vi "test Add-Import-Deploy.vi"(8 "error in":errorcluster, 11 "Import-Script-Deploy.lvclass":refnum<class "Import-Script-Deploy.lvclass">) -> (0 "error out":errorcluster, 3 "Import-Script-Deploy.lvclass":refnum<class "Import-Script-Deploy.lvclass">)   [LabVIEW 2020, in "Import-Script-Deploy.lvclass"]
uses:
  Import-Script-Deploy.lvclass
  C:/Git/niveristand-custom-device-testing-tools/VeriStandTestCase/VeriStandTestCase.lvclass
  Shared/Device Parameters.ctl
  Shared/Initialization Method.ctl
  Import-Script-Deploy.lvclass/Import-Script-Deploy.ctl
  4b06c685-66bb-4135-9ad1-d89a50a95502.vi
  <vilib>/addons/_JKI Toolkits/VI Tester/TestCase.llb/TestCase.lvclass
  Scripting/Ballard/Ballard ARINC 429 Scripting.lvlib
  niveristand-custom-device-testing-tools/VeriStandTestUtilities/VeriStandTestUtilities.lvlib
  C:/Program Files (x86)/National Instruments/LabVIEW 2020/vi.lib/addons/_JKI Toolkits/VI Tester/TestCase.llb/TestCase.lvclass
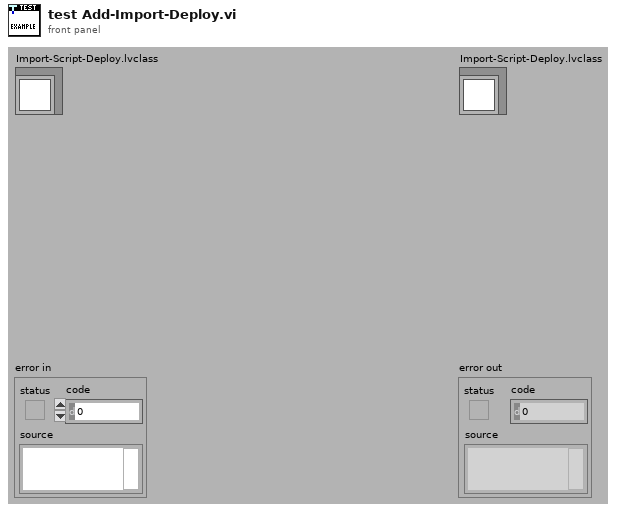
[diagram p1: front panel]
types:
  T1 = typedef "Device Parameters.ctl" = cluster{"initialization method":T2, "card number":i32, "PXI slot number":i32, "core number":i32}
  T2 = typedef "Initialization Method.ctl" = enum16{"PXI Slot Number", "Card Number"}
  T3 = typedef "Custom Device API.lvlib/Custom Device Item Ref.ctl" = u64
  T4 = typedef "NI_VS Workspace ExecutionAPI.lvlib/WorkspaceAPI.ctl" = refnum<k24>
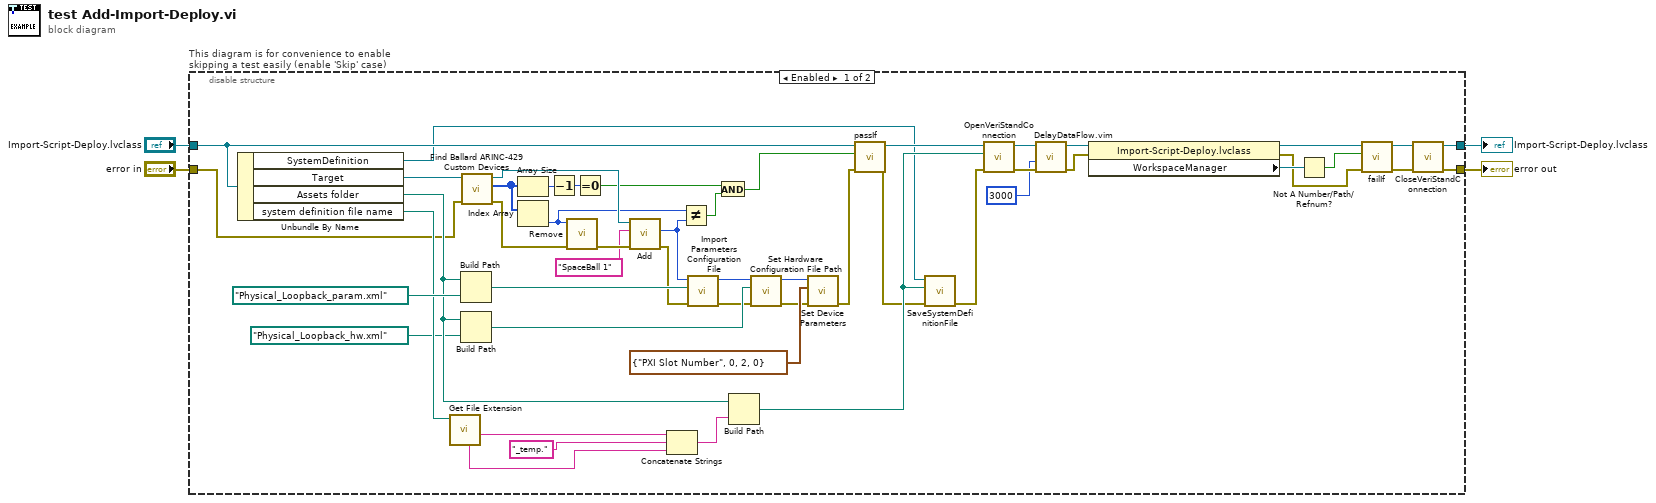
[diagram p0: block diagram]
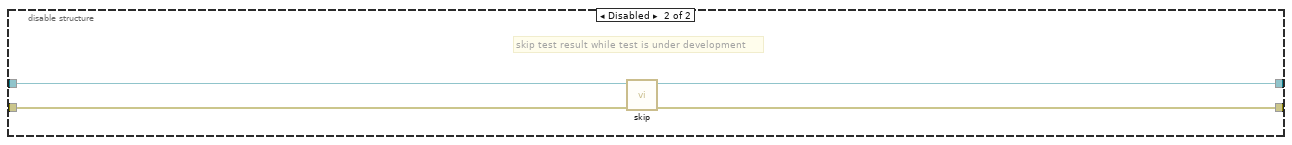
[diagram p2: hidden frame]
diagram:
  n1 = disable-structure "This diagram is for convenience to enable skipping a test easily (enable 'Skip' case)" shown="Enabled" {
    disable-tunnel: "Import-Script-Deploy.lvclass" -> [w43 w57]
    disable-tunnel: [w52 w56] -> w3
    disable-tunnel: "error in" -> [w21 w55]
    disable-tunnel: [w45 w54] -> w1
    frame Enabled {
      n2 = Unbundle By Name(w43) -> ("SystemDefinition"=w22:refnum<k24>, "Target"=w44:refnum<k24>, "Assets folder"=w28:path, "system definition file name"=w36:path)
      n3 = call <vilib>:"Get File Extension.vi"("file"=w36) -> ("filename without extension"=w35:string, "unmodified file extension"=w33:string)  [unwired: 6 in, 3 out]
      n4 = Build Path(base path=w28, name or relative path=path "Physical_Loopback_param.xml" ("Absolute or Relative Path")) -> (appended path=w18:path)
      n5 = Build Path(base path=w28, name or relative path=path "Physical_Loopback_hw.xml" ("Absolute or Relative Path")) -> (appended path=w26:path)
      n6 = call "Find Ballard ARINC-429 Custom Devices.vi"("error in"=w21, "target in"=w44) -> ("error out"=w13:errorcluster, "Ballard ARINC 429 custom devices"=w20:u64[], "target out"=w15:refnum<k24>)  [unwired: 7 in]
      n7 = Array Size(array=w20) -> (size(s)=w11:i32)
      n8 = Index Array(array=w20) -> (element=w8:u64)  [unwired: 1 in]
      n9 = Decrement(x=w11) -> (x-1=w10:i32)
      n10 = call "Remove.vi"("error in"=w13, "Ballard ARINC 429 custom device"=w8) -> ("error out"=w16:errorcluster)  [unwired: 9 in]
      n11 = Equal To 0?(x=w10) -> (x = 0?=w7:bool)
      n12 = call "Add.vi"("error in"=w16, "name"="SpaceBall 1", "target in"=w15) -> ("error out"=w12:errorcluster, "Ballard ARINC 429 ref out"=w9:T3)  [unwired: 6 in, 1 out]
      n13 = Concatenate Strings(w35, "_temp." ("string"), w33) -> (w32:string)
      n14 = Not Equal?(x=w8, y=w9) -> (x != y?=w6:bool)
      n15 = call "Import Parameters Configuration File.vi"("error in"=w12, "parameters configuration file path"=w18, "Ballard ARINC 429 ref"=w9) -> ("error out"=w17:errorcluster, "Ballard ARINC 429 ref out"=w19:T3)  [unwired: 7 in]
      n16 = And(x=w7, y=w6) -> (x .and. y?=w5:bool)
      n17 = Build Path(base path=w28, name or relative path=w32) -> (appended path=w31:path)
      n18 = call "Set Hardware Configuration File Path.vi"("error in"=w17, "path"=w26, "custom device ref"=w19) -> ("error out"=w24:errorcluster, "custom device ref out"=w25:T3)  [unwired: 7 in]
      n19 = call "Set Device Parameters.vi"("error in"=w24, "device parameters"=T1 {"initialization method"=enum."PXI Slot Number", "card number"=0, "PXI slot number"=2, "core number"=0}, "Ballard ARINC 429 custom device in"=w25) -> ("error out"=w23:errorcluster)  [unwired: 7 in, 1 out]
      n20 = call-dynamic "passIf.vi"("error in (no error)"=w23, "pass"=w5, "TestCase in"=w43) -> ("error out"=w29:errorcluster, "TestCase out"=w42:refnum<class "Import-Script-Deploy.lvclass">)  [unwired: 7 in]
      n21 = call "SaveSystemDefinitionFile.vi"("error in (no error)"=w29, "System Definition File in"=w31, "System Definition Reference in"=w22) -> ("error out"=w30:errorcluster)  [unwired: 7 in, 1 out]
      n22 = call-dynamic "OpenVeriStandConnection.vi"("error in (no error)"=w30, "System Definition File"=w31, "VeriStand Test Case in"=w42) -> ("error out"=w41:errorcluster, "VeriStand Test Case out"=w40:refnum<class "Import-Script-Deploy.lvclass">)  [unwired: 6 in, 1 out]
      n23 = call "DelayDataFlow.vim"("value in"=w41, "milliseconds to wait"=u32 3000) -> ("value out"=w53:errorcluster)  [unwired: 2 in, 1 out]
      n24 = property class="Import-Script-Deploy.lvclass"(reference=w40, error in=w53) -> (reference out=w51:refnum<class "Import-Script-Deploy.lvclass">, error out=w46:errorcluster, "WorkspaceManager"=w48:T4)
      n25 = Not A Number/Path/Refnum?(number/path/refnum=w48) -> (NaN/Path/Refnum?=w47:bool)
      n26 = call-dynamic "failIf.vi"("error in (no error)"=w46, "fail"=w47, "TestCase in"=w51) -> ("error out"=w49:errorcluster, "TestCase out"=w50:refnum<class "Import-Script-Deploy.lvclass">)  [unwired: 7 in]
      n27 = call-dynamic "CloseVeriStandConnection.vi"("error in (no error)"=w49, "VeriStand Test Case in"=w50) -> ("error out"=w52:errorcluster, "VeriStand Test Case out"=w45:refnum<class "Import-Script-Deploy.lvclass">)  [unwired: 8 in]
    }
    frame Disabled {
      # "skip test result while test is under development"
      n28 = call <vilib>:"skip.vi"("error in (no error)"=w55, "TestCase in"=w57) -> ("error out"=w56:errorcluster, "TestCase out"=w54:refnum<class "Import-Script-Deploy.lvclass">)  [unwired: 8 in]
    }
  }
  "error out" <- w3
  "Import-Script-Deploy.lvclass" <- w1
